vi "Error Converter (ErrCode or Status).vi"(8 "error in (no error)":errorcluster caption="错误输入（无错误）", 11 "error code":i32 caption="错误代码") -> (0 "error out":errorcluster caption="错误输出")   [LabVIEW 2024, in "GAS.lvlib"]
uses:
  GAS.lvlib
panel:
  in  "string":string="该错误由共享库函数返回。" caption="字符串"
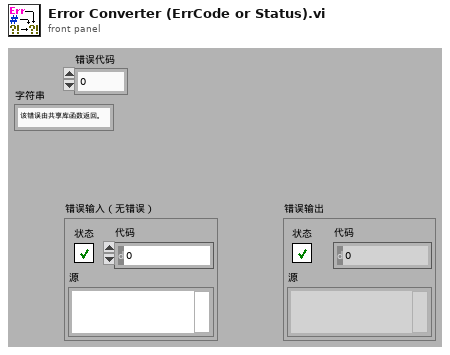
[diagram p1: front panel]
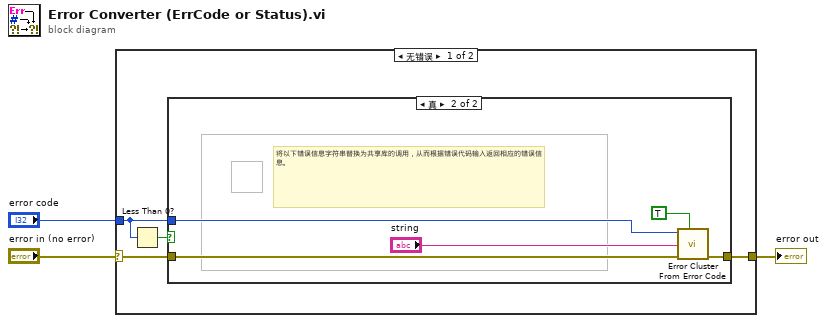
[diagram p0: block diagram]
diagram:
  n1 = case shown="无错误" "error in (no error)" {
    selector: "error in (no error)" -> [w6 w14]
    tunnel: [w4 w14] -> w2
    tunnel: "error code" -> [w5 _]
    frame No Error {
      n2 = Less Than 0?(x=w5) -> (x < 0?=w7:bool)
      n3 = case shown="真" w7 {
        tunnel: w6 -> [w8 w13]
        tunnel: w5 -> [_ w11]
        tunnel: [w8 w12] -> w4
        frame False {
        }
        frame True {
          # "将以下错误信息字符串替换为共享库的调用，从而根据错误代码输入返回相应的错误信息。"
          n4 = call <vilib>:"Error Cluster From Error Code.vi"("show call chain? (False)"=TRUE, "error in (no error)"=w13, "error message (\"\")"="string", "error code (0)"=w11) -> ("error out"=w12:errorcluster)  [unwired: 5 in]
        }
      }
    }
    frame Error {
    }
  }
  "error out" <- w2
